vi "ROI_Focus_test.vi"() -> ()   [LabVIEW 2014]
doc: "This VI is doing following things:\n1. select an ROI from the last image of the image sequence;\n2. use the selected 4 ROIs to calculate the focal plane coord."
uses:
  <vilib>/Utility/miscctls.llb/LVPoint32TypeDef.ctl
  <vilib>/Utility/miscctls.llb/LVPositionTypeDef.ctl
  <vilib>/Utility/miscctls.llb/LVBoundsTypeDef.ctl
  TypeDef/inputImages.ctl
panel:
  out "Draw Area Size":T1
  in  "Zoom Factor":sgl=0.3
  out "Selected image":picture
  out "top":i16
  out "bottom":i16
  out "left":i16
  out "right":i16
  out "PicOriginPosition":T2
  out "MouseUp":T3
  in  "Focus":bool
  out "MouseDown":T3
  out "Image":picture
  in  "Input_Z":dbl[](array[numeric])=[1.0, 2.0, 3.0, 4.0]
  out "Elapsed time (s)":dbl
  in  "Image4":path=path "C:/Users/light/Desktop/Peng/Raman/Images/3.png"
  in  "Image3":path=path "C:/Users/light/Desktop/Peng/Raman/Images/2.png"
  in  "Image2":path=path "C:/Users/light/Desktop/Peng/Raman/Images/1.png"
  out "BestPosition":dbl
  in  "Image1":path=path "C:/Users/light/Desktop/Peng/Raman/Images/0.png"
  # "This VI is doing following\nthings:\n1. select an ROI from the\nlast image of the image\nsequence;\n2. use the selected 4 ROIs\nto calculate the focal plane\ncoord."
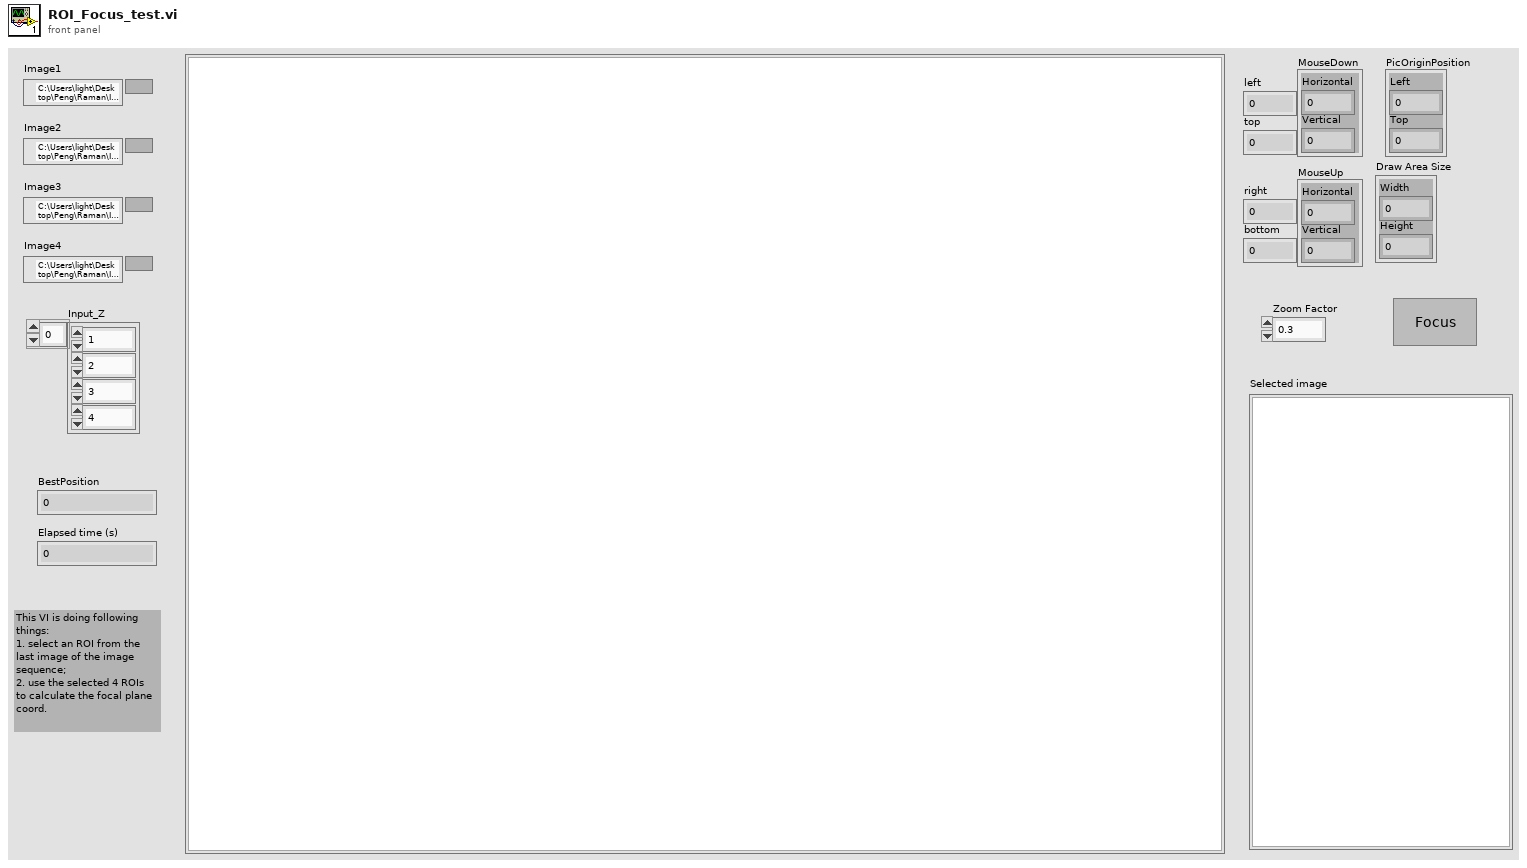
[diagram p1: front panel]
types:
  T1 = typedef "LVBoundsTypeDef.ctl" = cluster{"Width":u32, "Height":u32}
  T2 = typedef "LVPositionTypeDef.ctl" = cluster{"Left":i32, "Top":i32}
  T3 = typedef "LVPoint32TypeDef.ctl" = cluster{"Horizontal":i32, "Vertical":i32}
  T4 = cluster{"left":i16, "top":i16, "right":i16, "bottom":i16}
  T5 = typedef "imagedata.ctl" = cluster{"image type":i32, "image depth":i32, "image":u8[], "mask":u8[], "colors":u32[], "Rectangle":cluster{"left":i16, "top":i16, "right":i16, "bottom":i16}}
  T6 = typedef "inputImages.ctl" = cluster{"Image2":u8[][], "Image3":u8[][], "Image4":u8[][], "Image1":u8[][]}
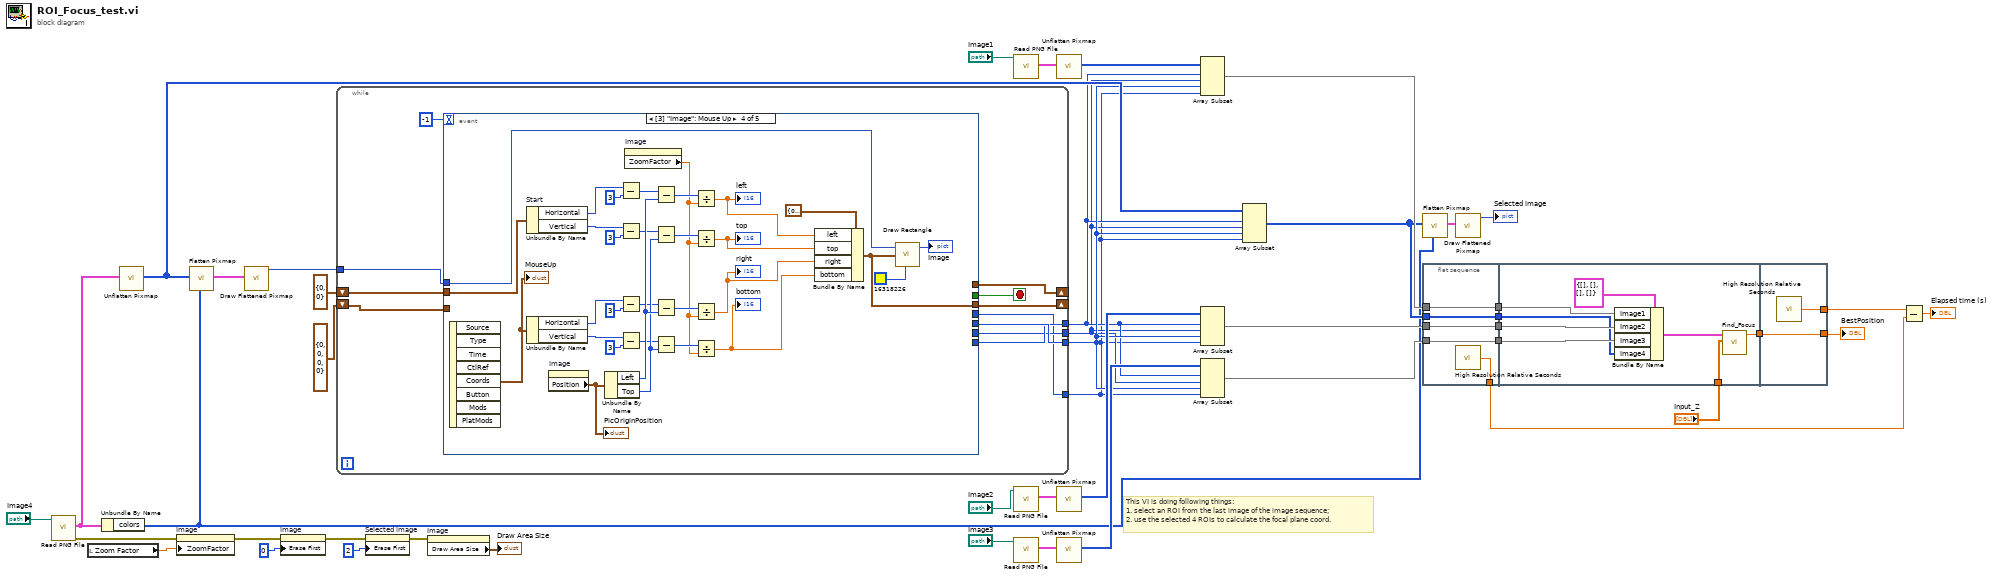
[diagram p0: block diagram]
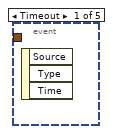
[diagram p2: hidden frame]
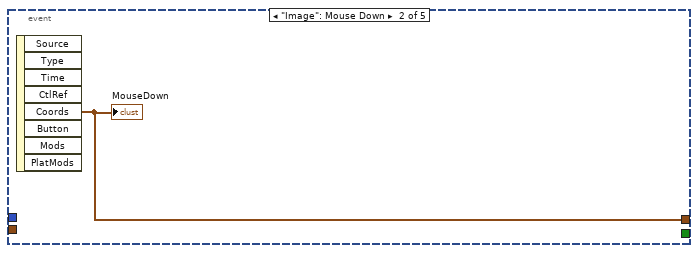
[diagram p3: hidden frame]
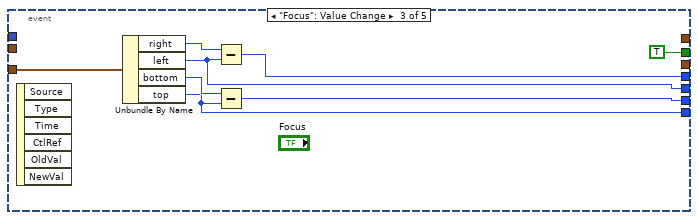
[diagram p4: hidden frame]
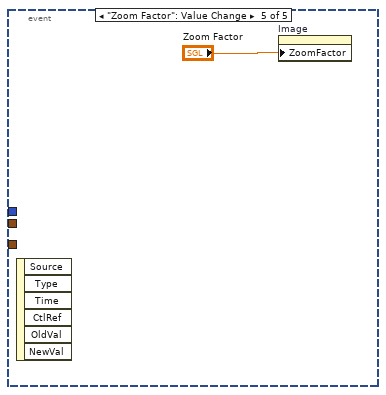
[diagram p5: hidden frame]
diagram:
  # "This VI is doing following things:\n1. select an ROI from the last image of the image sequence;\n2. use the selected 4 ROIs to calculate the focal plane coord."
  n1 = call <vilib>:"Read PNG File.vi"("path to PNG file"="Image4") -> ("error out"=w13:errorcluster, "image data"=w19:T5)  [unwired: 8 in, 1 out]
  n2 = local read "Zoom Factor"() -> (w4:sgl)
  n3 = Unbundle By Name(w19) -> ("colors"=w9:u32[])
  n4 = call <vilib>:"Unflatten Pixmap.vi"("image data"=w19) -> ("8-bit pixmap"=w18:u8[][])  [unwired: 4 in, 6 out]
  n5 = property on="Image" class="Pict"(error in=w13, "ZoomFactor"=w4) -> (error out=w7:errorcluster)  [unwired: 1 in, 1 out]
  n6 = call <vilib>:"Flatten Pixmap.vi"("colors"=w9, "8-bit pixmap"=w18) -> ("image data"=w24:T5)  [unwired: 9 in]
  n7 = call <vilib>:"Draw Flattened Pixmap.vi"("image data"=w24) -> ("new picture"=w20:picture)  [unwired: 8 in]
  n8 = property on="Image" class="Pict"(error in=w7, "Erase First"=u8 0) -> (error out=w6:errorcluster)  [unwired: 1 in, 1 out]
  n9 = while {
    shift-right: [w54] -> _
    shift-left: T3 {"Horizontal"=0, "Vertical"=0} ("Coords") -> [w53]
    tunnel: w20 -> [w52]
    shift-right: [w51] -> _
    shift-left: T4 {"left"=0, "top"=0, "right"=0, "bottom"=0} ("rect") -> [w50]
    tunnel: [w49] -> w17
    tunnel: [w48] -> w16
    tunnel: [w47] -> w15
    tunnel: [w46] -> w14
    stop <- w55 stop-if-true
    n10 = event shown="[3] \"Image\": Mouse Up" {
      selector: _ -> [_ _ _ _ _]
      dyn-events: _ -> [_ _ _ _ _]
      timeout: -1 -> [_ _ _ _ _]
      tunnel: [_ _ TRUE ("Stop") _ _] -> w55
      tunnel: [_ w57 _ _ _] -> w54
      tunnel: w53 -> [_ _ _ w96 _]
      tunnel: w52 -> [_ _ _ w93 _]
      tunnel: [_ _ _ w76 _] -> w51
      tunnel: w50 -> [_ _ w64 _ _]
      tunnel: [_ _ w61 _ _] -> w49
      tunnel: [_ _ w58 _ _] -> w48
      tunnel: [_ _ w60 _ _] -> w47
      tunnel: [_ _ w59 _ _] -> w46
      event Timeout {
        n11 = event-data() -> ()  [unwired: 1 in, 3 out]
      }
      event "Image": Mouse Down {
        n12 = event-data() -> ("Coords"=w57:T3)  [unwired: 1 in, 7 out]
        "MouseDown" <- w57
      }
      event "Focus": Value Change {
        n13 = event-data() -> ()  [unwired: 1 in, 6 out]
        n14 = Unbundle By Name(w64) -> ("right"=w62:i16, "left"=w61:i16, "bottom"=w63:i16, "top"=w58:i16)
        n15 = Subtract(x=w62, y=w61) -> (x-y=w59:i16)
        n16 = Subtract(x=w63, y=w58) -> (x-y=w60:i16)
      }
      event "Image": Mouse Up {
        n17 = event-data() -> ("Coords"=w95:T3)  [unwired: 1 in, 7 out]
        "MouseUp" <- w95
        n18 = Unbundle By Name "Start"(w96) -> ("Horizontal"=w89:i32, "Vertical"=w86:i32)
        n19 = Unbundle By Name(w95) -> ("Horizontal"=w83:i32, "Vertical"=w80:i32)
        n20 = property on="Image" class="Pict"() -> ("Position"=w90:T2)  [unwired: 2 in, 2 out]
        "PicOriginPosition" <- w90
        n21 = Unbundle By Name(w90) -> ("Left"=w92:i32, "Top"=w91:i32)
        n22 = Subtract(x=w89, y=3) -> (x-y=w87:i32)
        n23 = Subtract(x=w86, y=3) -> (x-y=w85:i32)
        n24 = Subtract(x=w83, y=3) -> (x-y=w81:i32)
        n25 = Subtract(x=w80, y=3) -> (x-y=w78:i32)
        n26 = property on="Image" class="Pict"() -> ("ZoomFactor"=w70:sgl)  [unwired: 2 in, 2 out]
        n27 = Subtract(x=w87, y=w92) -> (x-y=w74:i32)
        n28 = Subtract(x=w85, y=w91) -> (x-y=w73:i32)
        n29 = Subtract(x=w81, y=w92) -> (x-y=w72:i32)
        n30 = Subtract(x=w78, y=w91) -> (x-y=w71:i32)
        n31 = Divide(x=w74, y=w70) -> (x/y=w69:sgl)
        "left" <- w69
        n32 = Divide(x=w73, y=w70) -> (x/y=w68:sgl)
        "top" <- w68
        n33 = Divide(x=w72, y=w70) -> (x/y=w67:sgl)
        "right" <- w67
        n34 = Divide(x=w71, y=w70) -> (x/y=w66:sgl)
        "bottom" <- w66
        n35 = Bundle By Name(cluster=T4 {"left"=0, "top"=0, "right"=0, "bottom"=0} ("rect"), "left"=w69, "top"=w68, "right"=w67, "bottom"=w66) -> (w76:T4)
        n36 = call <vilib>:"Draw Rectangle.vi"("picture"=w93, "rect"=w76, "color(black)"=u32 16318226) -> ("new picture"=→"Image":picture)  [unwired: 6 in]
      }
      event "Zoom Factor": Value Change {
        n37 = event-data() -> ()  [unwired: 1 in, 6 out]
        n38 = property on="Image" class="Pict"("ZoomFactor"="Zoom Factor") -> ()  [unwired: 2 in, 2 out]
      }
    }
  }
  n39 = property on="Selected image" class="Pict"(error in=w6, "Erase First"=u8 2) -> (error out=w1:errorcluster)  [unwired: 1 in, 1 out]
  n40 = property on="Image" class="Pict"(error in=w1) -> ("Draw Area Size"=→"Draw Area Size":T1)  [unwired: 1 in, 2 out]
  n41 = call <vilib>:"Read PNG File.vi"("path to PNG file"="Image1") -> ("image data"=w22:T5)  [unwired: 8 in, 2 out]
  n42 = call <vilib>:"Read PNG File.vi"("path to PNG file"="Image2") -> ("image data"=w44:T5)  [unwired: 8 in, 2 out]
  n43 = call <vilib>:"Read PNG File.vi"("path to PNG file"="Image3") -> ("image data"=w41:T5)  [unwired: 8 in, 2 out]
  n44 = call <vilib>:"Unflatten Pixmap.vi"("image data"=w22) -> ("8-bit pixmap"=w25:u8[][])  [unwired: 4 in, 6 out]
  n45 = call <vilib>:"Unflatten Pixmap.vi"("image data"=w44) -> ("8-bit pixmap"=w29:u8[][])  [unwired: 4 in, 6 out]
  n46 = call <vilib>:"Unflatten Pixmap.vi"("image data"=w41) -> ("8-bit pixmap"=w27:u8[][])  [unwired: 4 in, 6 out]
  n47 = Array Subset(array=w25, index (row)=w16, length (row)=w15, index (col)=w17, length (col)=w14) -> (w23:u8[][])
  n48 = Array Subset(array=w29, index (row)=w16, length (row)=w15, index (col)=w17, length (col)=w14) -> (w28:u8[][])
  n49 = Array Subset(array=w27, index (row)=w16, length (row)=w15, index (col)=w17, length (col)=w14) -> (w26:u8[][])
  n50 = Array Subset(array=w18, index (row)=w16, length (row)=w15, index (col)=w17, length (col)=w14) -> (w11:u8[][])
  n51 = call <vilib>:"Flatten Pixmap.vi"("colors"=w9, "8-bit pixmap"=w11) -> ("image data"=w12:T5)  [unwired: 9 in]
  n52 = flat-sequence {
    tunnel: w11 -> [w99]
    tunnel: w26 -> [w100]
    tunnel: w28 -> [w101]
    tunnel: w23 -> [w102]
    tunnel: [w102] -> w37
    tunnel: [w101] -> w36
    tunnel: [w100] -> w35
    tunnel: [w99] -> w34
    tunnel: [w98] -> w31
    tunnel: [w110] -> w38
    tunnel: w37 -> [w108]
    tunnel: w36 -> [w107]
    tunnel: w35 -> [w106]
    tunnel: w34 -> [w105]
    tunnel: "Input_Z" -> [w103]
    tunnel: [w112] -> w39
    tunnel: w38 -> [w112]
    tunnel: [w111] -> w32
    frame #0 {
      n53 = call <vilib>:"High Resolution Relative Seconds.vi"() -> ("relative seconds"=w98:dbl)
    }
    frame #1 {
      n54 = Bundle By Name(cluster=T6 {"Image2"=[], "Image3"=[], "Image4"=[], "Image1"=[]} ("Imput images"), "Image1"=w108, "Image2"=w107, "Image3"=w106, "Image4"=w105) -> (w104:T6)
      n55 = call "Find_Focus.vi"("Input_Z"=w103, "Imput images"=w104) -> ("BestPosition"=w110:dbl)  [unwired: 8 in, 1 out]
    }
    frame #2 {
      n56 = call <vilib>:"High Resolution Relative Seconds.vi"() -> ("relative seconds"=w111:dbl)
    }
  }
  n57 = call <vilib>:"Draw Flattened Pixmap.vi"("image data"=w12) -> ("new picture"=→"Selected image":picture)  [unwired: 8 in]
  n58 = Subtract(x=w32, y=w31) -> (x-y=→"Elapsed time (s)":dbl)
  "BestPosition" <- w39
